vi "TIO Stream Open.vi"(7 "Port timeout":u32=500, 10 "Default baud":u32=115200, 11 "URL":refnum<visa-resource-name>="tcp://localhost") -> (0 "error out":errorcluster, 1 "Connected":bool=TRUE, 3 "TC Connection":T1={"Type"=enum."Serial", "URL"="serial:///dev/cu.usbserial-00000", "TO"=500, "Addr"=0, "Port"=0, "TCP"=refnum, "UDP"=refnum, "Route"=""})   [LabVIEW 2010]
uses:
  <vilib>/Utility/tcp.llb/UDP Multicast Read-Write Open.vi
  <vilib>/Instr/_visa.llb/VISA Configure Serial Port (Instr).vi
  <userlib>/TIO Library 2010/TIO Serial Port Discovery.vi
panel:
  in  "Default Port":i32=7855
  in  "error in (no error)":errorcluster
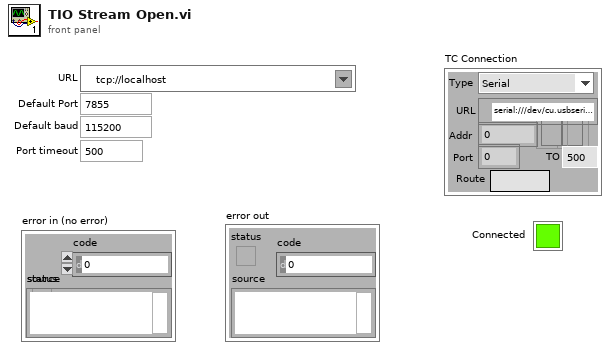
[diagram p1: front panel]
types:
  T1 = cluster{"Type":enum16{"Serial", "TCP", "UDP", "mUDP"}, "URL":refnum<visa-resource-name>, "TO":u32, "Addr":u32, "Port":i32, "TCP":refnum<k5>, "UDP":refnum<k16>, "Route":string}
  T2 = cluster{"Type":u16, "VISA resource name out":refnum<visa-resource-name>, "Port timeout":u32, u32, "Default Port":i32, "connection ID":refnum<k5>, "UDP":refnum<k16>, "string":string}
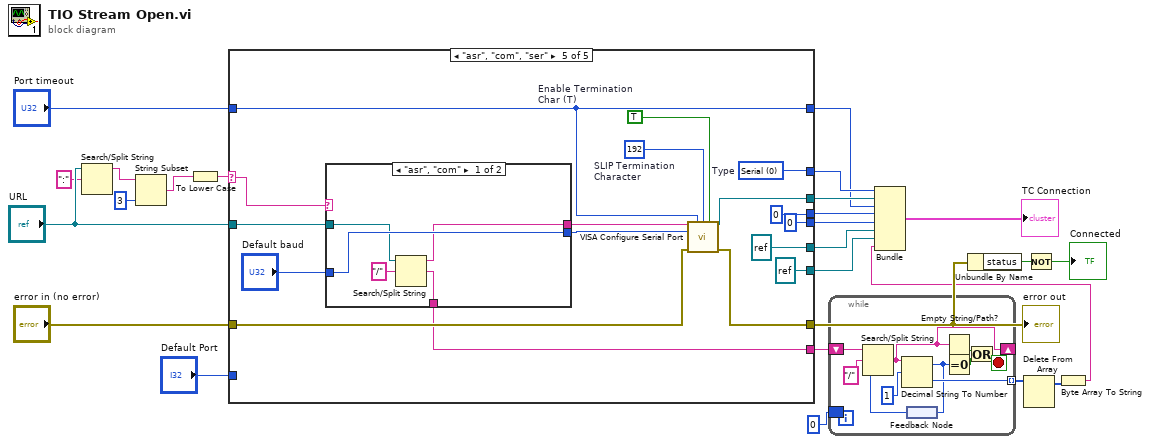
[diagram p0: block diagram]
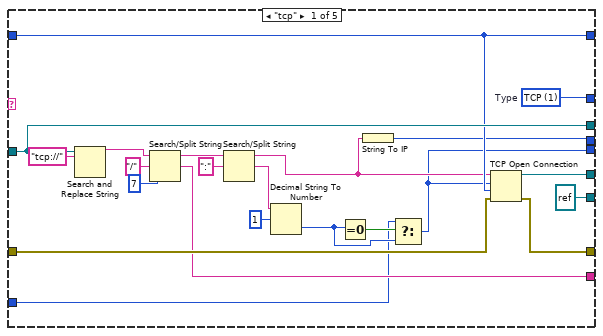
[diagram p2: hidden frame]
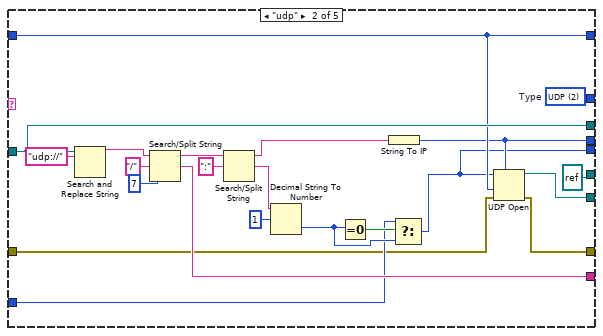
[diagram p3: hidden frame]
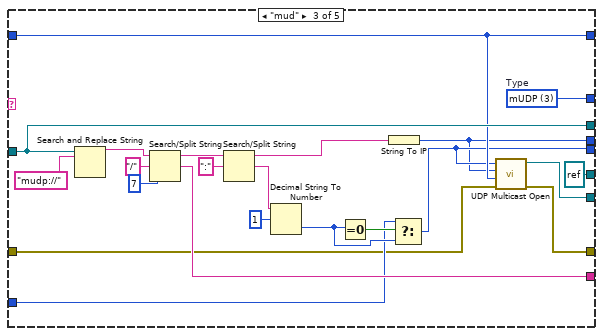
[diagram p4: hidden frame]
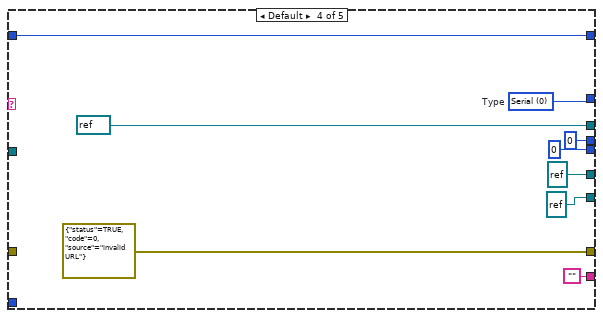
[diagram p5: hidden frame]
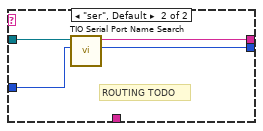
[diagram p6: hidden frame]
diagram:
  n1 = Search/Split String(string="URL", search string/char (-)=":") -> (substring before match=w23:string)  [unwired: 1 in, 2 out]
  n2 = String Subset(string=w23, length (rest)=3 ("length (rest)")) -> (substring=w20:string)  [unwired: 1 in]
  n3 = To Lower Case(string=w20) -> (all lower case string=w21:string)
  n4 = case shown="\"asr\", \"com\", \"ser\"" w21 {
    selector: w21 -> [_ _ _ _ w112]
    tunnel: [w40 w55 w74 errorcluster {"status"=TRUE, "code"=0, "source"="invalid URL"} ("error out") w111] -> w19
    tunnel: [w38 w63 w85 refnum<visa-resource-name> refnum ("VISA resource name out") w110] -> w14
    tunnel: "URL" -> [w38 w63 w85 _ w115]
    tunnel: "error in (no error)" -> [w41 w56 w75 _ w109]
    tunnel: [w39 refnum<k5> refnum ("connection ID") refnum<k5> refnum ("connection ID") refnum<k5> refnum ("connection ID") refnum<k5> refnum ("connection ID")] -> w4
    tunnel: [w26 w48 w84 w94 w101] -> w16
    tunnel: "Port timeout" -> [w37 w52 w72 w97 w106]
    tunnel: [w37 w52 w72 w97 w106] -> w7
    tunnel: [w32 w58 w79 "" w105] -> w12
    tunnel: "Default Port" -> [w31 w57 w78 _ _]
    tunnel: [refnum<k16> refnum ("UDP") w54 w73 refnum<k16> refnum ("UDP") refnum<k16> refnum ("UDP")] -> w3
    tunnel: [w28 w50 w70 u32 0 u32 0] -> w6
    tunnel: [w27 w49 w71 0 ("Default Port") 0 ("Default Port")] -> w5
    frame "tcp" {
      w26 = u16 1 items=["Serial", "TCP", "UDP", "mUDP"]  # Type
      n5 = Search and Replace String(input string=w38, search string="tcp://") -> (result string=w34:string)  [unwired: 6 in, 3 out]
      n6 = Search/Split String(string=w34, search string/char (-)="/", offset (0)=7) -> (substring before match=w33:string, match + rest of string=w32:string)  [unwired: 1 out]
      n7 = Search/Split String(string=w33, search string/char (-)=":") -> (substring before match=w29:string, match + rest of string=w45:string)  [unwired: 1 in, 1 out]
      n8 = Decimal String To Number(string=w45, offset=1) -> (number=w43:i32)  [unwired: 1 in, 1 out]
      n9 = Equal To 0?(x=w43) -> (x = 0?=w42:bool)
      n10 = String To IP(1:w29) -> (0:w28:u32)
      n11 = Select(t=w31, s=w42, f=w43) -> (s? t:f=w27:i32)
      n12 = TCP Open Connection(address=w29, remote port or service name=w27, timeout ms (60000)=w37, error in (no error)=w41) -> (connection ID=w39:refnum<k5>, error out=w40:errorcluster)  [unwired: 1 in]
    }
    frame "udp" {
      w48 = u16 2 items=["Serial", "TCP", "UDP", "mUDP"]  # Type
      n13 = Search and Replace String(input string=w63, search string="udp://") -> (result string=w60:string)  [unwired: 6 in, 3 out]
      n14 = Search/Split String(string=w60, search string/char (-)="/", offset (0)=7) -> (substring before match=w59:string, match + rest of string=w58:string)  [unwired: 1 out]
      n15 = Search/Split String(string=w59, search string/char (-)=":") -> (substring before match=w51:string, match + rest of string=w67:string)  [unwired: 1 in, 1 out]
      n16 = Decimal String To Number(string=w67, offset=1) -> (number=w65:i32)  [unwired: 1 in, 1 out]
      n17 = Equal To 0?(x=w65) -> (x = 0?=w64:bool)
      n18 = String To IP(1:w51) -> (0:w50:u32)
      n19 = Select(t=w57, s=w64, f=w65) -> (s? t:f=w49:i32)
      n20 = UDP Open(7:w50, 8:w56, 9:w52, 11:w49) -> (port=w54:refnum<k16>, 0:w55:errorcluster)  [unwired: 1 in, 1 out]
    }
    frame "mud" {
      w84 = u16 3 items=["Serial", "TCP", "UDP", "mUDP"]  # Type
      n21 = Search and Replace String(input string=w85, search string="mudp://") -> (result string=w81:string)  [unwired: 6 in, 3 out]
      n22 = Search/Split String(string=w81, search string/char (-)="/", offset (0)=7) -> (substring before match=w80:string, match + rest of string=w79:string)  [unwired: 1 out]
      n23 = Search/Split String(string=w80, search string/char (-)=":") -> (substring before match=w76:string, match + rest of string=w89:string)  [unwired: 1 in, 1 out]
      n24 = Decimal String To Number(string=w89, offset=1) -> (number=w87:i32)  [unwired: 1 in, 1 out]
      n25 = Equal To 0?(x=w87) -> (x = 0?=w86:bool)
      n26 = String To IP(1:w76) -> (0:w70:u32)
      n27 = Select(t=w78, s=w86, f=w87) -> (s? t:f=w71:i32)
      n28 = call-poly <vilib>:"UDP Multicast Open.vi"("error in (no error)"=w75, "time-to-live (1)"=w72, "multicast addr"=w70, "port"=w71) -> ("error out"=w74:errorcluster, "connection ID"=w73:refnum<k16>)  [unwired: 5 in, 1 out]
    }
    frame Default {
      w94 = u16 0 items=["Serial", "TCP", "UDP", "mUDP"]  # Type
    }
    frame "asr", "com", "ser" {
      w101 = u16 0 items=["Serial", "TCP", "UDP", "mUDP"]  # Type
      w116 = TRUE  # Enable Termination Char (T)
      w117 = u8 192  # SLIP Termination Character
      n29 = case shown="\"asr\", \"com\"" w112 {
        tunnel: w115 -> [w119 w126]
        tunnel: [w118 w125] -> w114
        tunnel: [w122 w124] -> w113
        tunnel: "Default baud" -> [w122 w123]
        tunnel: [w120 _] -> w105
        frame "asr", "com" {
          n30 = Search/Split String(string=w119, search string/char (-)="/") -> (substring before match=w118:string, match + rest of string=w120:string)  [unwired: 1 in, 1 out]
        }
        frame "ser", Default {
          # "ROUTING TODO"
          n31 = call <userlib>:"TIO Serial Port Name Search.vi"("Default baud"=w123, "String"=w126) -> ("Baud"=w124:i32, "VISA Resource"=w125:string)  [unwired: 7 in, 1 out]
        }
      }
      n32 = call-poly "VISA Configure Serial Port"("VISA resource name"=w114, "timeout (10sec)"=w106, "termination char\n(0xA = '\\n' = LF)"=w117, "Enable Termination\nChar (T)"=w116, "baud rate (9600)"=w113, "error in (no error)"=w109) -> ("VISA resource name out"=w110:refnum<visa-resource-name>, "error out"=w111:errorcluster)  [unwired: 8 in]
    }
  }
  "error out" <- w19
  n33 = while {
    tunnel: [w133] -> w11 mode=indexing
    shift-right: [w129] -> _
    shift-left: w12 -> [w135]
    border: 0 ("offset past number") -> [_]
    stop <- w130 stop-if-true
    n34 = feedback #1() -> (w127:i32)
    n35 = Search/Split String(string=w135, search string/char (-)="/", offset (0)=w127) -> (match + rest of string=w129:string)  [unwired: 2 out]
    n36 = Decimal String To Number(string=w129, offset=1) -> (offset past number=w128:i32, number=w133:i32)  [unwired: 1 in]
    n37 = feedback-in #1(w128) -> ()
    n38 = Empty String/Path?(string/path=w129) -> (empty?=w132:bool)
    n39 = Equal To 0?(x=w128) -> (x = 0?=w131:bool)
    n40 = Or(x=w132, y=w131) -> (x .or. y?=w130:bool)
  }
  n41 = Unbundle By Name(w19) -> ("status"=w18:bool)
  n42 = Delete From Array(array=w11) -> (array with subset deleted=w10:i32[])  [unwired: 2 in, 1 out]
  n43 = Not(x=w18) -> (.not. x?=→"Connected":bool)
  n44 = Byte Array To String(unsigned byte array=w10) -> (string=w2:string)
  n45 = Bundle("Type"=w16, "VISA resource name out"=w14, "Port timeout"=w7, w6, "Default Port"=w5, "connection ID"=w4, "UDP"=w3, "string"=w2) -> (→"TC Connection":T2)  [unwired: 1 in]
